vi "MathOptim-Sigmoid Model.vi"(3 "output control":T1, 4 "data":variant, 5 "X":dbl[](array[numeric]), 6 "a":dbl[](array[numeric])) -> (0 "error out":errorcluster, 1 "f'(X,a)":dbl[][](array[numeric]), 2 "f(X,a)":dbl[](array[numeric]))   [LabVIEW 2020]
doc: "This template is the starting point for creating a model function to be passed to the Nonlinear Curve Fit.vi."
uses:
  <vilib>/gmath/NumericalOptimization/LM_output select.ctl
  <vilib>/Analysis/7linalg.llb/Solve Linear Equations (single right hand).vi
  <vilib>/Analysis/baseanly.llb/Solve Linear Equations By Cholesky.vi
  <vilib>/Analysis/baseanly.llb/Real Matrix to Compact Array.vi
  <vilib>/Analysis/baseanly.llb/Real Compact Tri-Matrix Linear Eqs.vi
  <vilib>/Analysis/7linalg.llb/Solve Linear Eqs (General).vi
  <vilib>/Analysis/7linalg.llb/Solve Linear Eqs (Gen, single right hand).vi
  <vilib>/Analysis/NI_AALPro.lvlib
  <vilib>/gmath/NI_Gmath.lvlib
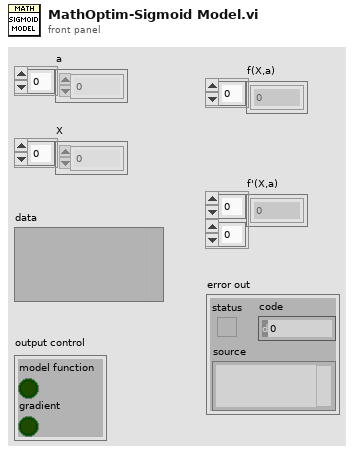
[diagram p1: front panel]
types:
  T1 = typedef "NI_Gmath.lvlib/LM_output select.ctl" = cluster{"model function":bool, "gradient":bool}
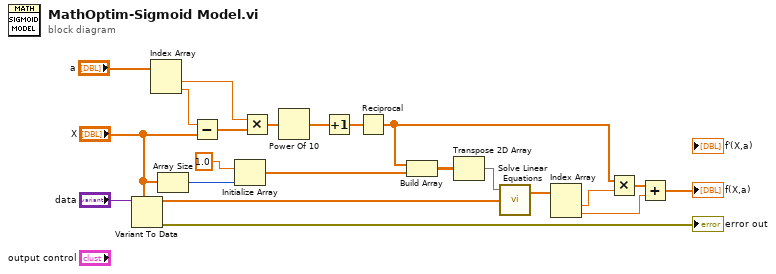
[diagram p0: block diagram]
diagram:
  n1 = Variant To Data(type="X", Variant="data") -> (data=w19:dbl[], error out=→"error out":errorcluster)  [unwired: 1 in]
  n2 = Index Array(array="a") -> (element #1=w4:dbl, element #2=w6:dbl)  [unwired: 2 in]
  n3 = Array Size(array="X") -> (size(s)=w18:i32)
  n4 = Subtract(x=w6, y="X") -> (x-y=w3:dbl[])
  n5 = Initialize Array(1.0, w18) -> (w16:dbl[])
  n6 = Multiply(x=w4, y=w3) -> (x*y=w2:dbl[])
  n7 = Power Of 10(x=w2) -> (10^x=w1:dbl[])
  n8 = Increment(x=w1) -> (x+1=w8:dbl[])
  n9 = Reciprocal(x=w8) -> (1/x=w7:dbl[])
  n10 = Build Array(w7, w16) -> (w15:dbl[][])
  n11 = Transpose 2D Array(2D array=w15) -> (transposed array=w9:dbl[][])
  n12 = call-poly <vilib>:"Solve Linear Equations.vi"("Known Vector"=w19, "Input Matrix"=w9) -> ("Solution Vector"=w14:dbl[])  [unwired: 1 in, 1 out]
  n13 = Index Array(array=w14) -> (element #1=w13:dbl, element #2=w11:dbl)  [unwired: 2 in]
  n14 = Multiply(x=w7, y=w13) -> (x*y=w12:dbl[])
  n15 = Add(x=w12, y=w11) -> (x+y=→"f(X,a)":dbl[])
